vi "Read CustomNikon.vi"(8 "error in (no error)":errorcluster, 11 "Nikon in":refnum<class "Nikon.lvclass">) -> (0 "error out":errorcluster, 2 "CustomNikon":string, 3 "Nikon out":refnum<class "Nikon.lvclass">)   [LabVIEW 2021, in "Nikon.lvclass"]
uses:
  Nikon.lvclass
  Nikon.lvclass/Nikon.ctl
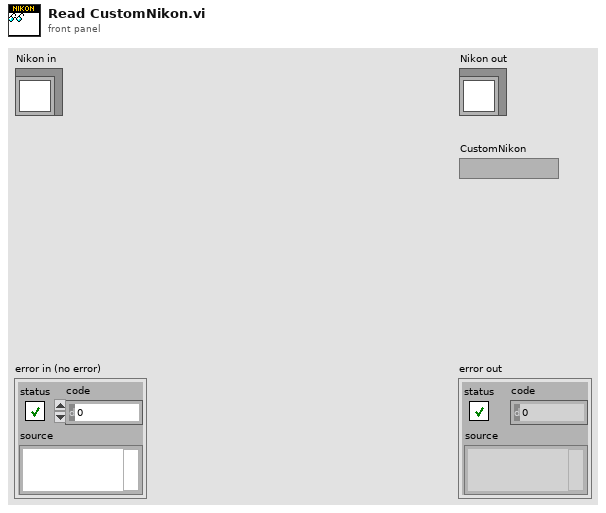
[diagram p1: front panel]
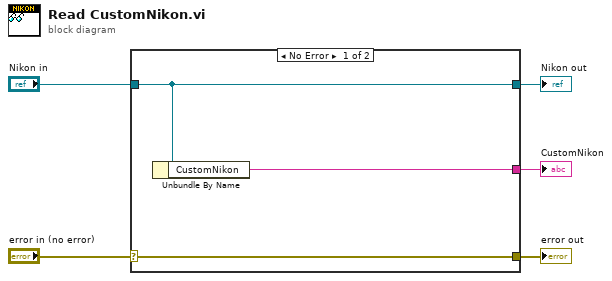
[diagram p0: block diagram]
diagram:
  n1 = case shown="No Error" "error in (no error)" {
    selector: "error in (no error)" -> [w8 w9]
    tunnel: [w8 w9] -> w4
    tunnel: [w7 w10] -> w2
    tunnel: "Nikon in" -> [w7 w10]
    tunnel: [w6 _] -> w1
    frame No Error {
      n2 = Unbundle By Name(w7) -> ("CustomNikon"=w6:string)
    }
    frame Error {
    }
  }
  "error out" <- w4
  "Nikon out" <- w2
  "CustomNikon" <- w1
